vi "Variant to Alarm Limits.vi"(8 "error in":errorcluster, 11 "value":variant) -> (0 "error out":errorcluster, 1 "alarm limits":T1={"Active"=FALSE, "Low Alarm Limit"=0.0, "Low Warning Limit"=0.0, "High Warning Limit"=0.0, "High Alarm Limit"=0.0, "Low Alarm Severity"=enum."major", "Low Warning Severity"=enum."minor", "High Warning Severity "=enum."minor", "High Alarm Severity"=enum."major", "Hysteresis"=0.0}, 2 "found?":bool, 3 "value out":variant)   [LabVIEW 2020, in "Value.lvlib"]
uses:
  Value.lvlib
  Alarm Limits.ctl
  Alarm Severity.ctl
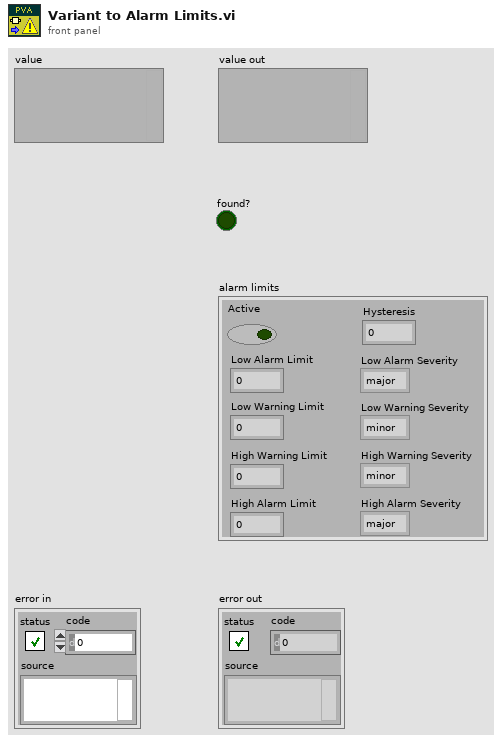
[diagram p1: front panel]
types:
  T1 = typedef "Value.lvlib/Alarm Limits.ctl" = cluster{"Active":bool, "Low Alarm Limit":dbl, "Low Warning Limit":dbl, "High Warning Limit":dbl, "High Alarm Limit":dbl, "Low Alarm Severity":T2, "Low Warning Severity":T2, "High Warning Severity ":T2, "High Alarm Severity":T2, "Hysteresis":dbl}
  T2 = typedef "Value.lvlib/Alarm Severity.ctl" = enum32{"no", "minor", "major", "record", "invalid", "undefined", ""}
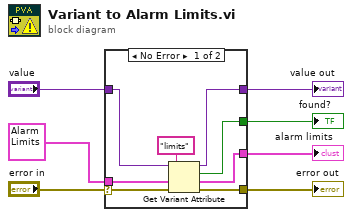
[diagram p0: block diagram]
diagram:
  n1 = case shown="No Error" "error in" {
    selector: "error in" -> [w14 w17]
    tunnel: [w11 w17] -> w7
    tunnel: "value" -> [w13 w16]
    tunnel: [w12 w16] -> w4
    tunnel: [w9 _] -> w1
    tunnel: T1 {"Active"=FALSE, "Low Alarm Limit"=0.0, "Low Warning Limit"=0.0, "High Warning Limit"=0.0, "High Alarm Limit"=0.0, "Low Alarm Severity"=enum."major", "Low Warning Severity"=enum."minor", "High Warning Severity "=enum."minor", "High Alarm Severity"=enum."major", "Hysteresis"=0.0} ("Alarm Limits") -> [w10 _]
    tunnel: [w8 _] -> w3
    frame No Error {
      n2 = Get Variant Attribute(Variant=w13, name="limits", default value (empty Variant)=w10, error in=w14) -> (duplicate Variant=w12:variant, found=w8:bool, value=w9:T1, error out=w11:errorcluster)
    }
    frame Error {
    }
  }
  "error out" <- w7
  "value out" <- w4
  "found?" <- w3
  "alarm limits" <- w1
